vi "Fixture PlugIn Configuration Dialog.vi"(10 "Automated Mode in":bool, 11 "Sequence Context":T1) -> (2 "Automated Mode out":bool)   [LabVIEW 2013]
doc: "Configure settings for the Test Fixture Plugin"
uses:
  <vilib>/addons/TestStand/_TSLegacy.llb/LabVIEW Test - Sequence Context.ctl
  <vilib>/addons/TestStand/_TSUtility.llb/TestStand - Start Modal Dialog (Sequence Context).vi
  <vilib>/addons/TestStand/_TSUtility.llb/TestStand - End Modal Dialog (Sequence Context).vi
  <vilib>/addons/TestStand/_TSUtility.llb/TestStand - Set Property Value (String).vi
panel:
  out "error out":errorcluster
  in  "OK":bool
  # "Use this plugin to configure the behavior of the test fixture.  The fixture supports automated UUT fixturing, which allows the test to execute multiple UUTs with no user interaction. When"
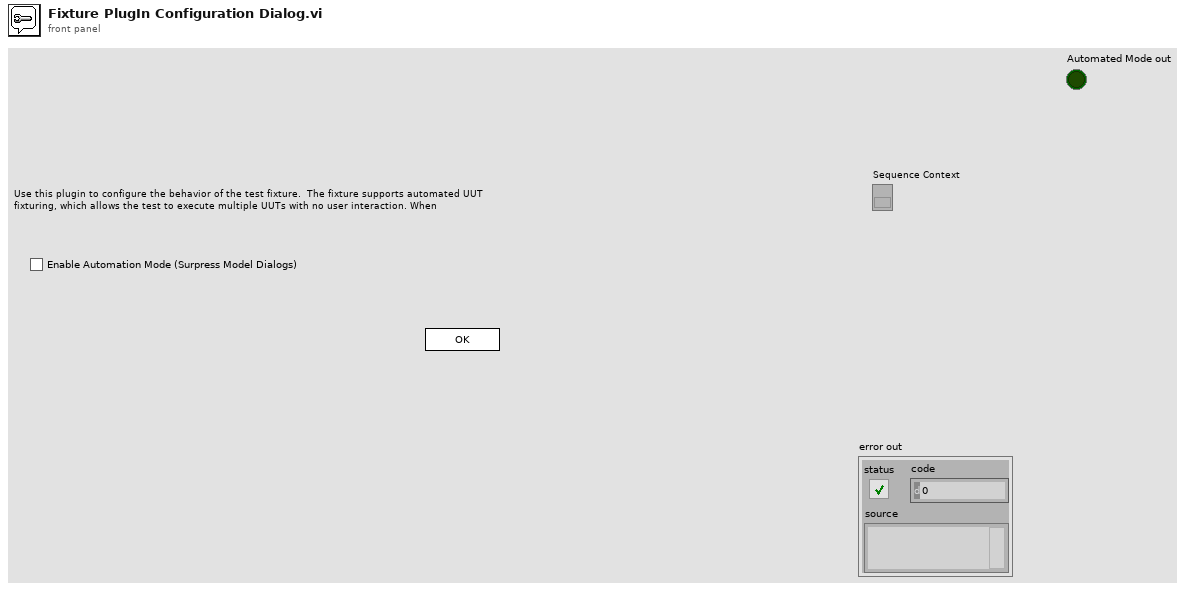
[diagram p1: front panel]
types:
  T1 = typedef "LabVIEW Test - Sequence Context.ctl" = refnum<k7>
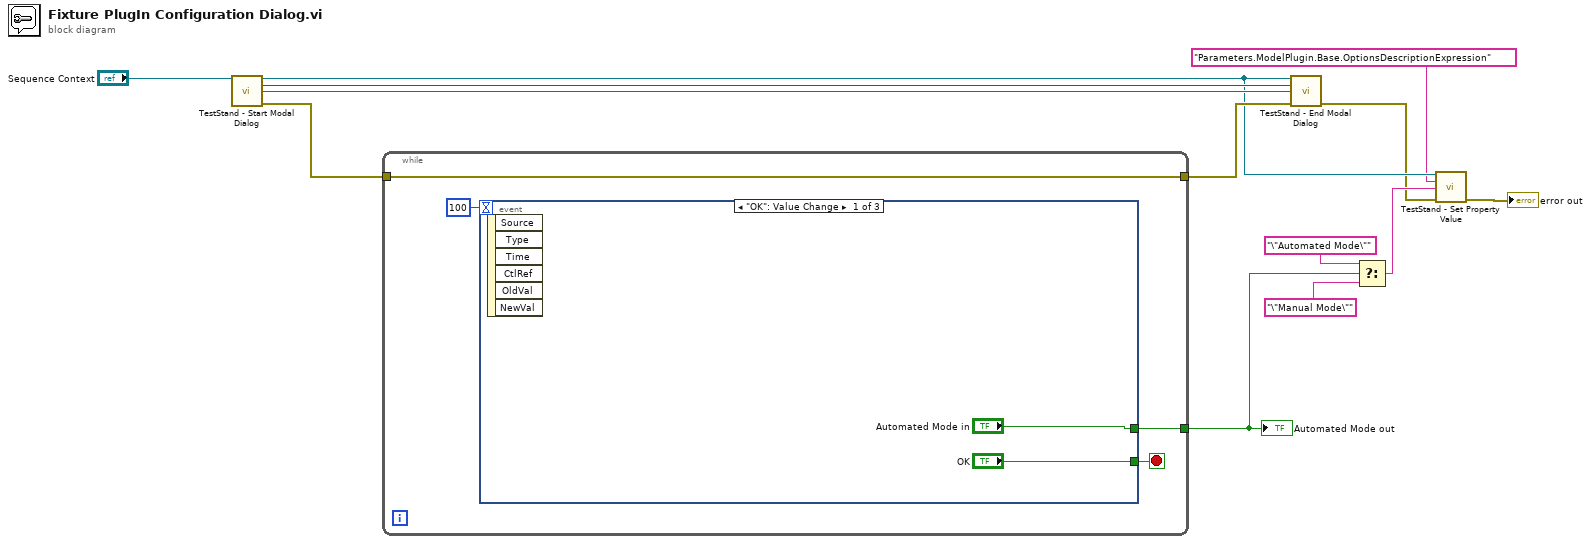
[diagram p0: block diagram]
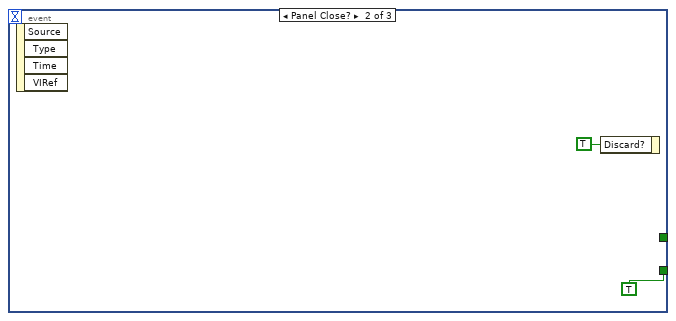
[diagram p2: hidden frame]
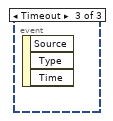
[diagram p3: hidden frame]
diagram:
  n1 = call-poly <vilib>:"TestStand - Start Modal Dialog.vi"("Sequence Context In"="Sequence Context") -> ("Sequence Context Out"=w5:refnum<k7>, "Modal ID"=w12:i32, "VI Originally Open"=w11:bool, "error out"=w1:errorcluster)  [unwired: 10 in, 1 out]
  n2 = while {
    tunnel: [w15] -> w9
    tunnel: [w14] -> w10
    tunnel: w1 -> [w14]
    stop <- w17 stop-if-true
    n3 = event shown="[0] \"OK\": Value Change" {
      selector: _ -> [_ _ _]
      dyn-events: _ -> [_ _ _]
      timeout: 100 -> [_ _ _]
      tunnel: ["OK" TRUE ("OK") _] -> w17
      tunnel: ["Automated Mode in" _ _] -> w15
      event "OK": Value Change {
        n4 = event-data() -> ()  [unwired: 1 in, 6 out]
      }
      event Panel Close? {
        n5 = event-data() -> ()  [unwired: 1 in, 4 out]
        n6 = event-data("Discard?"=TRUE) -> ()  [unwired: 1 in, 1 out]
      }
      event Timeout {
        n7 = event-data() -> ()  [unwired: 1 in, 3 out]
      }
    }
  }
  "Automated Mode out" <- w9
  n8 = call-poly <vilib>:"TestStand - End Modal Dialog.vi"("Sequence Context In"=w5, "Modal ID"=w12, "VI Originally Open"=w11, "error in (no error)"=w10) -> ("error out"=w4:errorcluster)  [unwired: 11 in]
  n9 = Select(t="\"Automated Mode\"", s=w9, f="\"Manual Mode\"") -> (s? t:f=w6:string)
  n10 = call-poly <vilib>:"TestStand - Set Property Value.vi"("Sequence Context In"=w5, "Lookup String"="Parameters.ModelPlugin.Base.OptionsDescriptionExpression", "New Value"=w6, "error in (no error)"=w4) -> ("error out"=→"error out":errorcluster)  [unwired: 10 in, 1 out]
